vi "Clear Target Faults.vi"(8 "error in (no error)":errorcluster, 10 "Clear Alarms":bool, 11 "Fault Monitor in":refnum<class "Fault Monitor.lvclass">) -> (0 "error out":errorcluster, 3 "Fault Monitor out":refnum<class "Fault Monitor.lvclass">)   [LabVIEW 2023, in "Fault Monitor.lvlib" / "Fault Monitor.lvclass"]
uses:
  Library/Fault Monitor.lvclass
  Custom Controls/Fault Map.ctl
  Library/Fault Monitor.lvclass/Fault Monitor.ctl
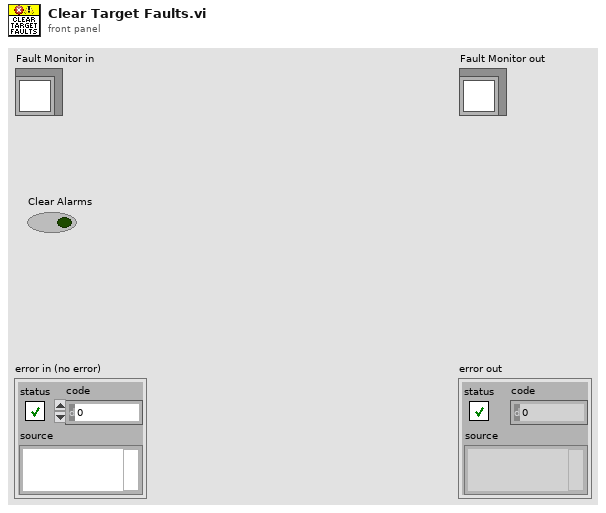
[diagram p1: front panel]
types:
  T1 = typedef "Fault Monitor.lvlib/Fault Monitor.lvclass/Fault Map.ctl" = map{string, errorcluster[]}
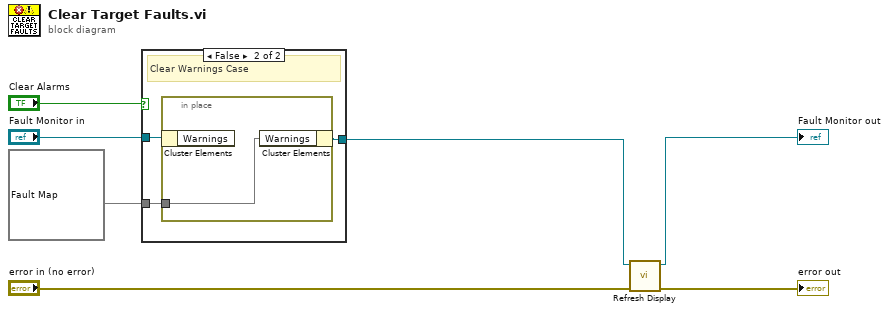
[diagram p0: block diagram]
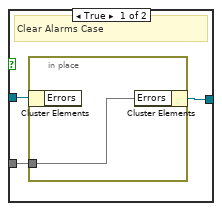
[diagram p2: hidden frame]
diagram:
  n1 = case shown="False" "Clear Alarms" {
    tunnel: "Fault Monitor in" -> [w10 w14]
    tunnel: [w9 w13] -> w5
    tunnel: T1 {} ("Errors") -> [w8 w12]
    frame True {
      # "Clear Alarms Case"
      n2 = in-place {
        in-place-border: w8 -> [w11]
        n3 = in-place-cluster #1(w10) -> ()  [unwired: 1 out]
        n4 = in-place-cluster #1("Errors"=w11) -> (w9:refnum<class "Fault Monitor.lvclass">)
      }
    }
    frame False {
      # "Clear Warnings Case"
      n5 = in-place {
        in-place-border: w12 -> [w15]
        n6 = in-place-cluster #2(w14) -> ()  [unwired: 1 out]
        n7 = in-place-cluster #2("Warnings"=w15) -> (w13:refnum<class "Fault Monitor.lvclass">)
      }
    }
  }
  n8 = call "Refresh Display.vi"("error in (no error)"="error in (no error)", "Fault Monitor in"=w5) -> ("error out"=→"error out":errorcluster, "Fault Monitor out"=→"Fault Monitor out":refnum<class "Fault Monitor.lvclass">)  [unwired: 8 in]
